vi "SetUser.vi"(8 "error in":errorcluster, 10 "User":string, 11 "OperationRun in":refnum<class "OperationRun.lvclass">) -> (0 "error out":errorcluster, 3 "OperationRun out":refnum<class "OperationRun.lvclass">)   [LabVIEW 2021, in "ProligentXMLGenerator.lvlib" / "OperationRun.lvclass"]
doc: "Defines the user that executed the operation run.\n\nThis value is limited to 255 charactesrs and must no be empty."
uses:
  OperationRun.lvclass
  OperationRun.lvclass/OperationRun.ctl
  Base/Attribute/Attribute.lvclass
  Base/NonEmptyString_255/NonEmptyString_255.lvclass
  C:/Projects/proligent-xml-generator-labview/src/ProligentXMLGenerator/Base/NonEmptyString/NonEmptyString.lvclass
  C:/Projects/proligent-xml-generator-labview/src/ProligentXMLGenerator/Base/String/String.lvclass
  C:/Projects/proligent-xml-generator-labview/src/ProligentXMLGenerator/Base/Attribute/Attribute.lvclass
  C:/Projects/proligent-xml-generator-labview/src/ProligentXMLGenerator/Base/NonEmptyString_255/NonEmptyString_255.lvclass
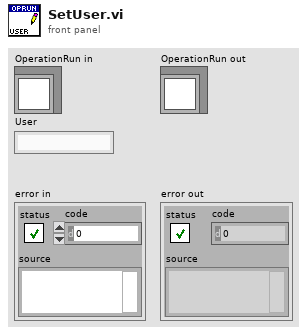
[diagram p1: front panel]
types:
  T1 = typedef "ProligentXMLGenerator.lvlib/OperationRun.lvclass/Data.ctl" = cluster{"Name":string, "Characteristics":refnum<class "Characteristic.lvclass">[], "Documents":refnum<class "Document.lvclass">[], "SequenceRuns":refnum<class "SequenceRun.lvclass">[], "FailureReferences":refnum<class "FailureReference.lvclass">[], "SequenceRunReferences":refnum<class "SequenceRunReference.lvclass">[], "CustomData":refnum<class "CustomData.lvclass">, "OperationRunId":refnum<class "Guid.lvclass">, "ProcessFullName":refnum<class "ProcessFullName.lvclass">, "ProcessVersion":refnum<class "NonEmptyString_64.lvclass">, "OperationName":refnum<class "NonEmptyString_65.lvclass">, "StationFullName":refnum<class "FullName.lvclass">, "User":refnum<class "NonEmptyString_255.lvclass">, "CallingOperationRunId":refnum<class "Guid.lvclass">, "OperationStatus":refnum<class "ExecutionStatus.lvclass">, "OperationRunStartTime":refnum<class "DateTime.lvclass">, "OperationRunEndTime":refnum<class "DateTime.lvclass">, "TimeZoneInfoId":string}
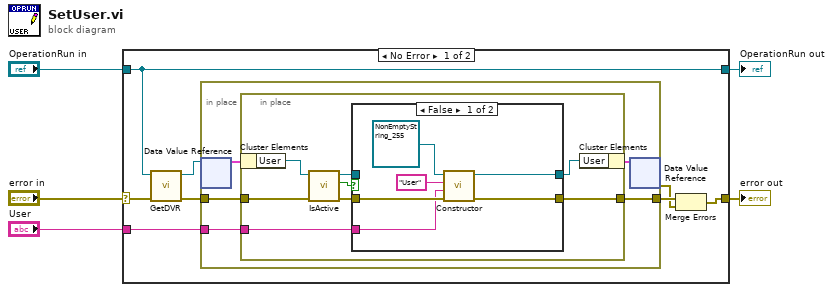
[diagram p0: block diagram]
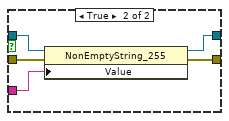
[diagram p2: hidden frame]
diagram:
  n1 = case shown="No Error" "error in" {
    selector: "error in" -> [w12 w38]
    tunnel: "OperationRun in" -> [w7 w39]
    tunnel: [w9 w38] -> w3
    tunnel: "User" -> [w8 _]
    tunnel: [w7 w39] -> w1
    frame No Error {
      n2 = call "GetDVR.vi"("error in"=w12, "OperationRun"=w7) -> ("error out"=w11:errorcluster, "DVRReference"=w13:refnum<data-value>)  [unwired: 8 in]
      n3 = in-place "In Place Element Structure" {
        in-place-border: w11 -> [w16]
        in-place-border: [w18] -> w10
        in-place-border: w8 -> [w17]
        n4 = in-place-dvr #1(w13) -> (w15:T1)  [unwired: 1 out]
        n5 = in-place "In Place Element Structure" {
          in-place-border: [w26] -> w18
          in-place-border: w17 -> [w25]
          in-place-border: w16 -> [w19]
          n6 = in-place-cluster #2(w15) -> ("User"=w24:refnum<class "NonEmptyString_255.lvclass">)
          n7 = call "IsActive.vi"("error in"=w19, "Attribute in"=w24) -> ("error out"=w22:errorcluster, "IsActive"=w20:bool, "Attribute in"=w21:refnum<class "NonEmptyString_255.lvclass">)  [unwired: 7 in]
          n8 = case shown="False" w20 {
            tunnel: [w31 w37] -> w26
            tunnel: w25 -> [w28 w36]
            tunnel: w22 -> [w32 w35]
            tunnel: w21 -> [_ w34]
            tunnel: [w27 w33] -> w23
            frame False {
              n9 = call-dynamic "Constructor.vi"("error in"=w32, "Value"=w28, "Name"="User", "String in"=refnum<class "NonEmptyString_255.lvclass"> refnum ("ProligentResultProcessor:NonEmptyString_255")) -> ("error out"=w31:errorcluster, "String out"=w27:refnum<class "NonEmptyString_255.lvclass">)  [unwired: 6 in]
            }
            frame True {
              n10 = property on="Property Node" class="NonEmptyString_255"(reference=w34, error in=w35, "Value"=w36) -> (reference out=w33:refnum<class "NonEmptyString_255.lvclass">, error out=w37:errorcluster)
            }
          }
          n11 = in-place-cluster #2("User"=w23) -> (w14:T1)
        }
        n12 = in-place-dvr #1(w14) -> (w6:errorcluster)  [unwired: 1 out]
      }
      n13 = Merge Errors(w10, w6) -> (w9:errorcluster)
    }
    frame Error {
    }
  }
  "error out" <- w3
  "OperationRun out" <- w1
